vi "Function generator.vi"() -> ()   [LabVIEW 2020]
uses:
  <vilib>/express/express analysis/Spectral/Block/exnSpectralBlock spectral measurements peak poly.vi
  <vilib>/express/express analysis/Spectral/Block/exnSpectralBlock spectral measurements peak DDT.vi
  <vilib>/express/express analysis/Spectral/XNode/ExpressSpectralMeasurementsBlockNode.xnode
panel:
  in  "Select signal":enum32{"sine", "square", "saw", "triangle"}(radio)
  out "TIME":dynamicdata(graph)
  out "Spectrm":dynamicdata(graph)
  in  "stop":bool
  in  "Phase":dbl
  in  "Offset":dbl
  in  "Freq":dbl=10.1 caption="Frequency"
  in  "Ampilitude":dbl=1.0 caption="Amplitude"
  # "1st button : sine \n2nd : square\n3rd : saw\n4th : triangle"
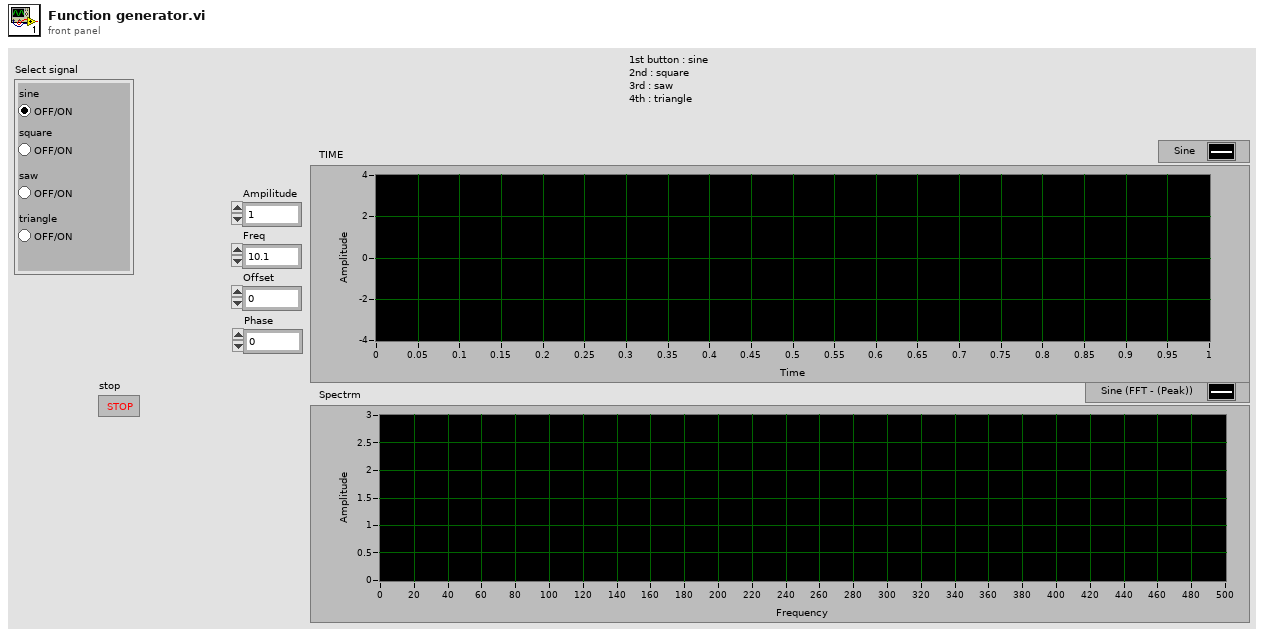
[diagram p1: front panel]
types:
  T1 = cluster{"averaging mode":u16, "weighting mode":u16, "number of averages":u32}
  T2 = cluster{"dB On (F)":bool, "unwrap phase (F)":bool, "convert to degree (F)":bool}
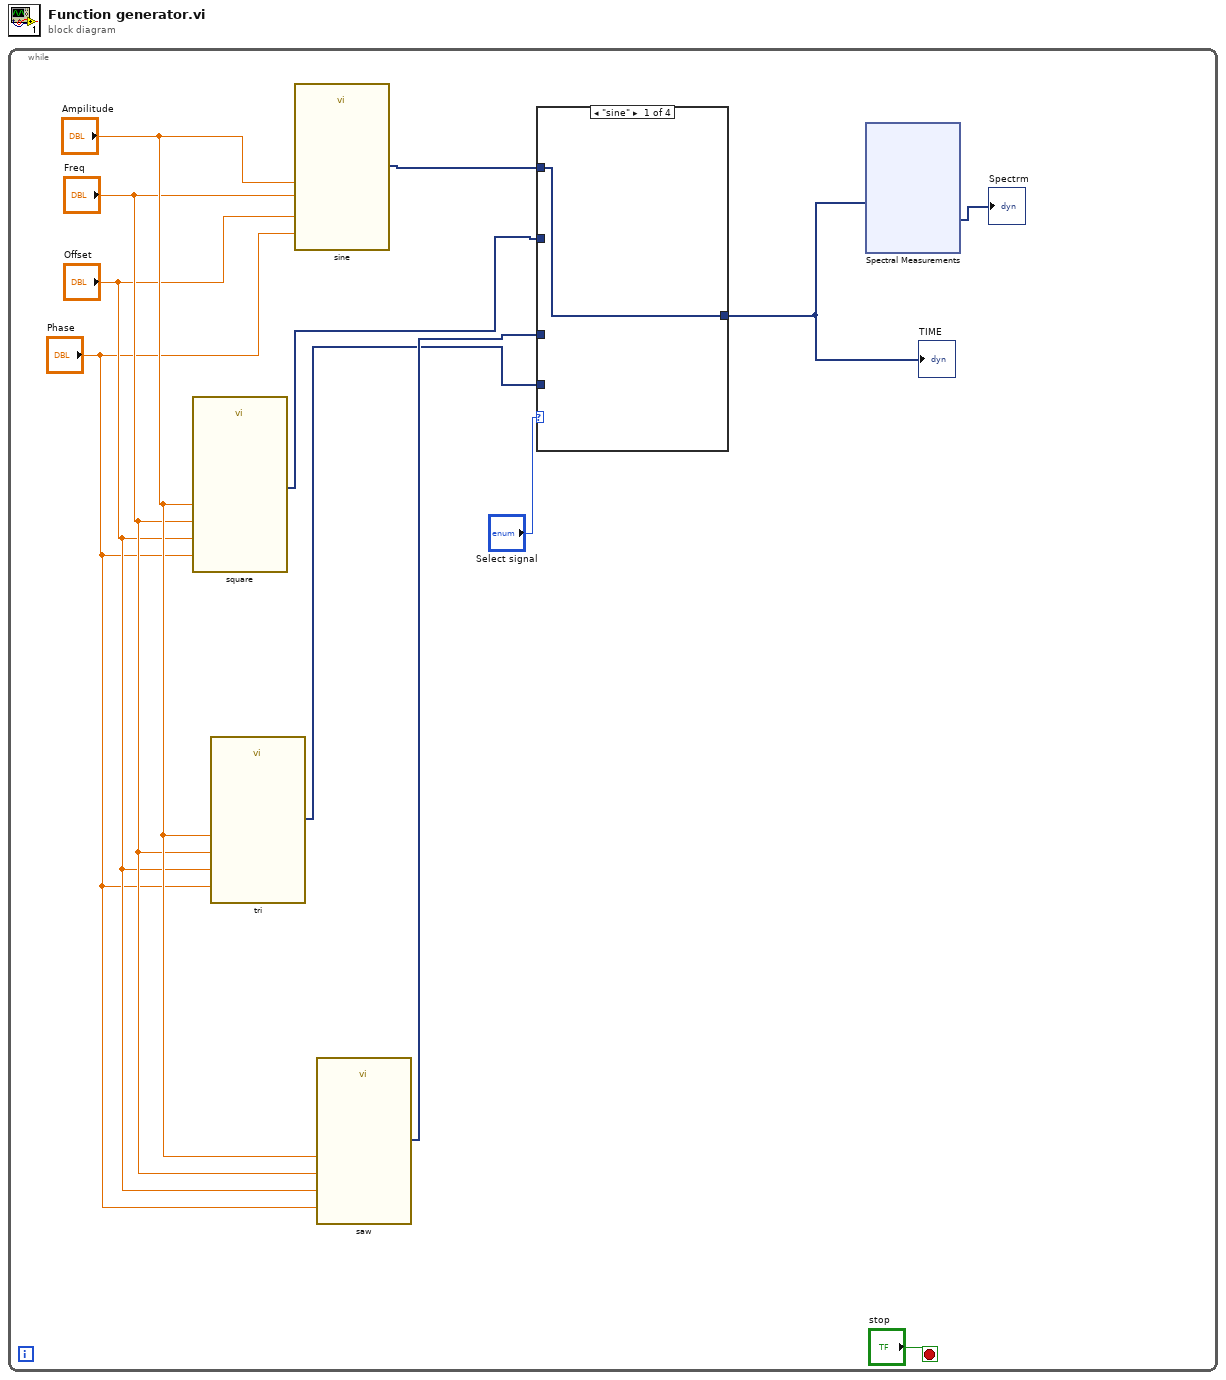
[diagram p0: block diagram]
diagram:
  n1 = while {
    stop <- "stop" stop-if-true
    n2 = call "square"("Offset"="Offset", "Frequency"="Freq", "Amplitude"="Ampilitude", "Phase"="Phase") -> ("Square"=w5:dynamicdata)  [unwired: 10 in, 1 out]
    n3 = call "tri"("Offset"="Offset", "Frequency"="Freq", "Amplitude"="Ampilitude", "Phase"="Phase") -> ("Triangle"=w3:dynamicdata)  [unwired: 10 in, 1 out]
    n4 = call "sine"("Offset"="Offset", "Frequency"="Freq", "Amplitude"="Ampilitude", "Phase"="Phase") -> ("Sine"=w6:dynamicdata)  [unwired: 10 in, 1 out]
    n5 = call "saw"("Offset"="Offset", "Frequency"="Freq", "Amplitude"="Ampilitude", "Phase"="Phase") -> ("Sawtooth"=w4:dynamicdata)  [unwired: 10 in, 1 out]
    n6 = case shown="\"sine\"" "Select signal" {
      tunnel: [w13 w14 w15 w16] -> w1
      tunnel: w6 -> [w13 _ _ _]
      tunnel: w5 -> [_ _ _ w16]
      tunnel: w4 -> [_ w14 _ _]
      tunnel: w3 -> [_ _ w15 _]
      frame "sine" {
      }
      frame "saw" {
      }
      frame "triangle" {
      }
      frame "square" {
      }
    }
    "TIME" <- w1
    n7 = xnode "Spectral Measurements"("Signals"=w1) -> ("FFT - (Peak)"=→"Spectrm":dynamicdata)  [unwired: 1 in, 2 out]
  }
